vi "离线通道使能(慢速).vi"(8 "错误输入":errorcluster caption="输出簇", 11 "文件句柄":i32) -> (0 "错误输出":errorcluster, 1 "通道数量":i32, 2 "AD通道使能":bool[](array[boolean]), 3 "文件句柄出":i32)   [LabVIEW 2011]
uses:
  dll/em9636.dll
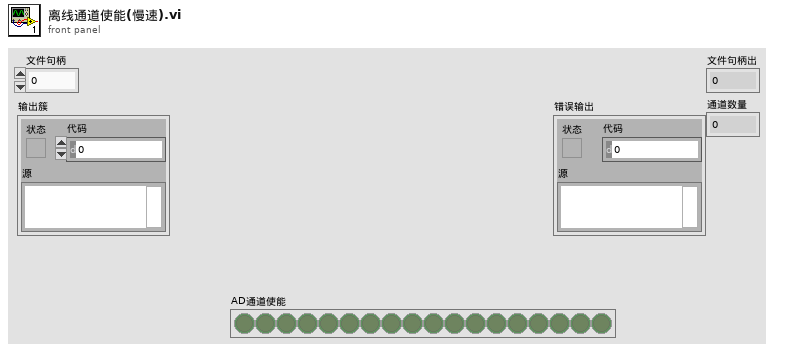
[diagram p1: front panel]
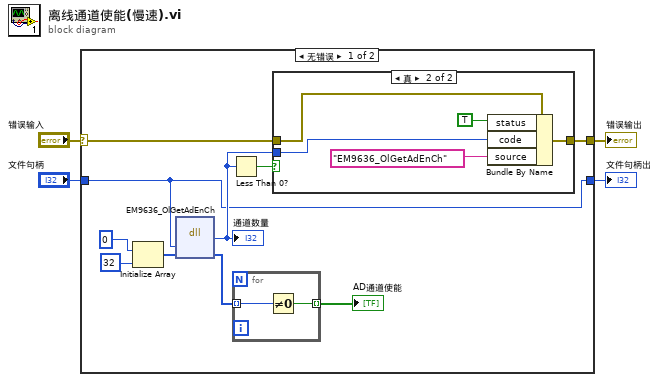
[diagram p0: block diagram]
diagram:
  n1 = case shown="无错误" "错误输入" {
    selector: "错误输入" -> [w5 w24]
    tunnel: [w7 w24] -> w3
    tunnel: "文件句柄" -> [w6 w23]
    tunnel: [w6 w23] -> w1
    frame No Error {
      n2 = Initialize Array(i8 0 ("元素"), 32 ("维数大小")) -> (w9:i8[])
      n3 = dll-call lib="PTH1abs Eèµ éç LABVIEWæºVI(v2.0)EM9636BD)EM9636BDè°ç¨APIå½æ°æ¹æ³éè®¯ä¾ç¨EM9636_demo_labview2011dll\nem9636.dll" fn="EM9636_OlGetAdEnCh"("文件句柄"=w6, "使能数组"=w9) -> ("通道数量"=w13:i32, "使能数组"=w12:i8[])  [unwired: 4 in, 2 out]
      "通道数量" <- w13
      n4 = Less Than 0?(x=w13) -> (x < 0?=w14:bool)
      n5 = for {
        tunnel: w12 -> [w16] mode=indexing
        tunnel: [w15] -> w8 mode=indexing
        n6 = Not Equal To 0?(x=w16) -> (x != 0?=w15:bool)
      }
      "AD通道使能" <- w8
      n7 = case shown="真" w14 {
        tunnel: [w17 w20] -> w7
        tunnel: w5 -> [w17 w22]
        tunnel: w13 -> [_ w19]
        frame False {
        }
        frame True {
          n8 = Bundle By Name(cluster=w22, "status"=TRUE, "code"=w19, "source"="EM9636_OlGetAdEnCh") -> (w20:errorcluster)
        }
      }
    }
    frame Error {
    }
  }
  "文件句柄出" <- w1
  "错误输出" <- w3
